vi "BuildCommCluster.vi"(6 "reply body":string, 7 "Type":string="GET", 8 "reply headers":string, 9 "sent body":string, 10 "sent headers":string, 11 "url":string) -> (3 "Comm":T1)   [LabVIEW 2022 SP3]
uses:
  HTTPComm.ctl
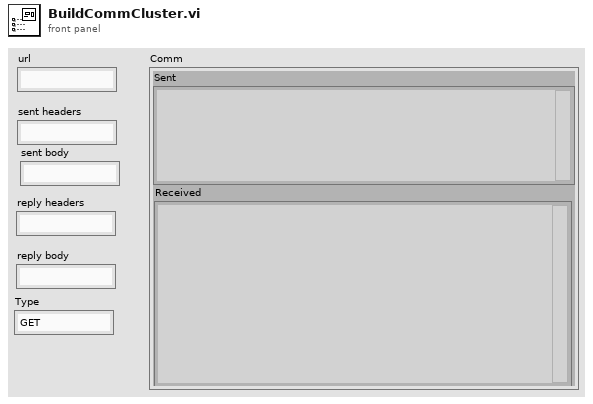
[diagram p1: front panel]
types:
  T1 = typedef "HTTPComm.ctl" = cluster{"url":string, "sent headers":string, "sent body":string, "headers":string, "body":string, "Sent":string, "Received":string}
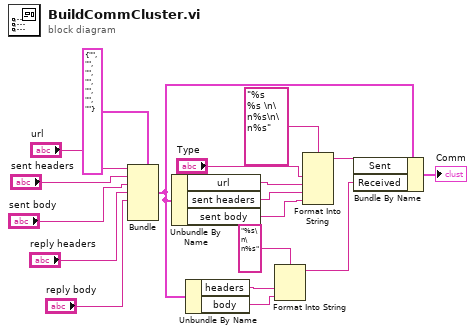
[diagram p0: block diagram]
diagram:
  n1 = Bundle(cluster=T1 {"url"="", "sent headers"="", "sent body"="", "headers"="", "body"="", "Sent"="", "Received"=""} ("Comm"), "url"="url", "sent headers"="sent headers", "sent body"="sent body", "headers"="reply headers", "body"="reply body") -> (w15:T1)  [unwired: 2 in]
  n2 = Unbundle By Name(w15) -> ("url"=w11:string, "sent headers"=w12:string, "sent body"=w2:string)
  n3 = Unbundle By Name(w15) -> ("headers"=w13:string, "body"=w14:string)
  n4 = Format Into String(format string="%s\n\n%s", w13, w14) -> (resulting string=w17:string)  [unwired: 2 in, 1 out]
  n5 = Format Into String(format string="%s %s \n\n%s\n\n%s", "Type", w11, w12, w2) -> (resulting string=w16:string)  [unwired: 2 in, 1 out]
  n6 = Bundle By Name(cluster=w15, "Sent"=w16, "Received"=w17) -> (→"Comm":T1)
